vi "Acquire.vi"(8 "error in (no error)":errorcluster, 9 "Data Queue":refnum<queue>, 10 "Data Notifier":refnum<notifier>, 11 "Hardware Resources in":T1={"DO"={"task name"="AI", "task_ref"="", "lines"=""}}) -> (0 "error out":errorcluster, 3 "Hardware Resources out":T1={"DO"={"task name"="AI", "task_ref"="", "lines"=""}})   [LabVIEW 2014]
doc: "Perform the acquisition. Replace the contents of this diagram with calls to acquisition hardware."
uses:
  <vilib>/Analysis/NI_AALBase.lvlib
  <vilib>/DAQmx/read.llb/DAQmx Read (Analog 1D Wfm NChan NSamp).vi
  GLB_compteurs.vi
  PLS Digital Control.lvlib
  <vilib>/DAQmx/read.llb/DAQmx Read (Counter DBL 1Chan 1Samp).vi
  GLB_AIs.vi
  Hardware Configuration.ctl
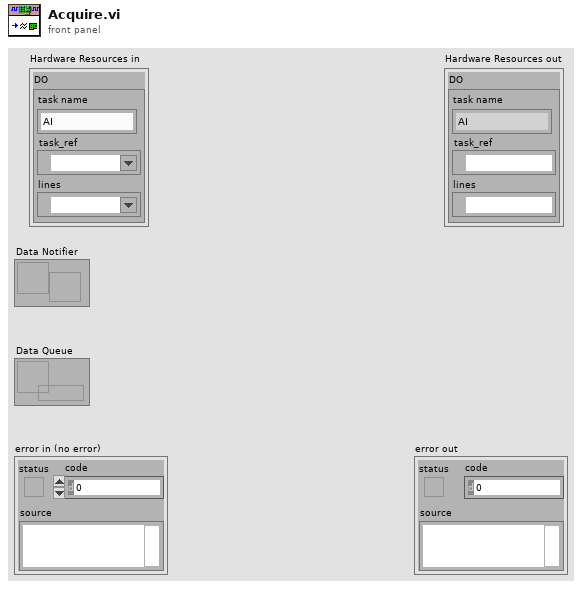
[diagram p1: front panel]
types:
  T1 = typedef "PLS Digital Control.lvlib/Hardware Configuration.ctl" = cluster{"DO":cluster{"task name":string, "task_ref":refnum<k21>, "lines":tag}}
  T2 = typedef "PLS Settings.lvlib/conversion.ctl" = cluster{"a":dbl, "b":dbl}
  T3 = cluster{"ai0":T2, "ai1":T2, "ai2":T2, "ai3":T2, "ai4":T2}
  T4 = cluster{"task name":string, "task_ref":refnum<k21>, "ctr":tag, "coeff":dbl}
  T5 = cluster{"[0]":dbl, "[1]":dbl, "[2]":dbl, "[3]":dbl, "[4]":dbl}
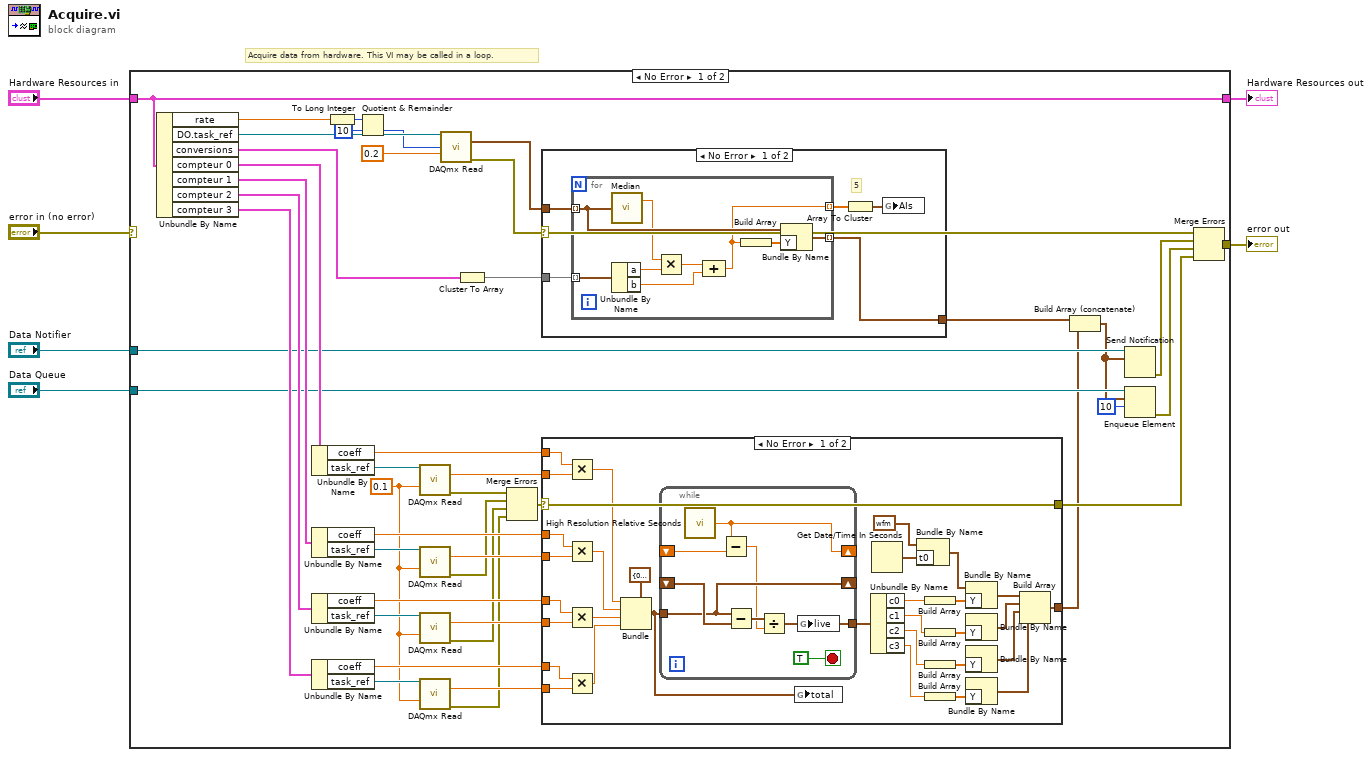
[diagram p0: block diagram]
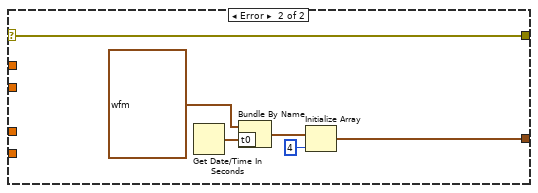
[diagram p2: hidden frame]
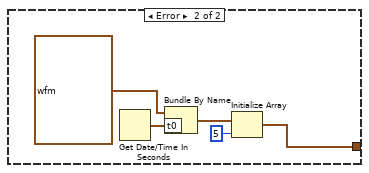
[diagram p3: hidden frame]
diagram:
  # "Acquire data from hardware. This VI may be called in a loop."
  n1 = case shown="No Error" "error in (no error)" {
    selector: "error in (no error)" -> [_ w115]
    tunnel: [w40 w115] -> w5
    tunnel: "Hardware Resources in" -> [w43 w116]
    tunnel: [w43 w116] -> w3
    tunnel: "Data Notifier" -> [w14 _]
    tunnel: "Data Queue" -> [w15 _]
    frame No Error {
      w20 = 0.1 ("timeout")
      n2 = Unbundle By Name(w43) -> ("rate"=w22:dbl, "DO.task_ref"=w49:refnum<k21>, "conversions"=w45:T3, "compteur 0"=w36:T4, "compteur 1"=w31:T4, "compteur 2"=w32:T4, "compteur 3"=w33:T4)
      n3 = Unbundle By Name(w36) -> ("coeff"=w34:dbl, "task_ref"=w35:refnum<k21>)
      n4 = Unbundle By Name(w31) -> ("coeff"=w29:dbl, "task_ref"=w30:refnum<k21>)
      n5 = Unbundle By Name(w32) -> ("coeff"=w27:dbl, "task_ref"=w28:refnum<k21>)
      n6 = Unbundle By Name(w33) -> ("coeff"=w25:dbl, "task_ref"=w26:refnum<k21>)
      n7 = To Long Integer(number=w22) -> (32bit integer=w21:i32)
      n8 = Quotient & Remainder(x=w21, y=10 ("number of samples per channel")) -> (floor(x/y)=w23:i32)  [unwired: 1 out]
      n9 = call-poly <vilib>:"DAQmx Read.vi"("task/channels in"=w35, "timeout"=w20) -> ("data"=w42:dbl, "error out"=w41:errorcluster)  [unwired: 11 in, 1 out]
      n10 = call-poly <vilib>:"DAQmx Read.vi"("task/channels in"=w30, "timeout"=w20) -> ("data"=w37:dbl, "error out"=w18:errorcluster)  [unwired: 11 in, 1 out]
      n11 = call-poly <vilib>:"DAQmx Read.vi"("task/channels in"=w28, "timeout"=w20) -> ("data"=w38:dbl, "error out"=w17:errorcluster)  [unwired: 11 in, 1 out]
      n12 = call-poly <vilib>:"DAQmx Read.vi"("task/channels in"=w26, "timeout"=w20) -> ("data"=w39:dbl, "error out"=w16:errorcluster)  [unwired: 11 in, 1 out]
      n13 = call-poly <vilib>:"DAQmx Read.vi"("task/channels in"=w49, "number of samples per channel"=w23, "timeout"=0.2) -> ("data"=w47:waveform(dbl)[], "error out"=w46:errorcluster)  [unwired: 10 in, 1 out]
      n14 = Cluster To Array(cluster=w45) -> (array=w44:T2[])
      n15 = Merge Errors(w41, w18, w17, w16) -> (w19:errorcluster)
      n16 = case shown="No Error" w46 {
        tunnel: w47 -> [w100 _]
        tunnel: w44 -> [w99 _]
        tunnel: [w96 w110] -> w13
        frame No Error {
          # "5"
          n17 = for {
            tunnel: w100 -> [w109] mode=indexing
            tunnel: [w108] -> w96 mode=indexing
            tunnel: w99 -> [w107] mode=indexing
            tunnel: [w101] -> w98 mode=indexing
            n18 = call <vilib>:"Median.vi"("X"=w109) -> ("median"=w105:dbl)  [unwired: 1 out]
            n19 = Unbundle By Name(w107) -> ("a"=w106:dbl, "b"=w103:dbl)
            n20 = Multiply(x=w105, y=w106) -> (x*y=w104:dbl)
            n21 = Compound Arithmetic op=ADD(w104, w103) -> (w101:dbl)
            n22 = Build Array(w101) -> (w102:dbl[])
            n23 = Bundle By Name(cluster=w109, "Y"=w102) -> (w108:waveform(dbl))
          }
          n24 = Array To Cluster(array=w98) -> (cluster=w97:T5)
          n25 = global write "GLB_AIs.vi" "AIs"(w97) -> ()
        }
        frame Error {
          n26 = Get Date/Time In Seconds() -> (seconds since 1Jan1904=w114:timestamp)
          n27 = Bundle By Name(cluster=waveform(dbl) {"t0"=timestamp(0 s since 1904-01-01), "dt"=0.1, "Y"=[nan]} ("waveform"), "t0"=w114) -> (w112:waveform(dbl))
          n28 = Initialize Array(w112, 5 ("dimension size")) -> (w110:waveform(dbl)[])
        }
      }
      n29 = case shown="No Error" w19 {
        selector: w19 -> [w80 w95]
        tunnel: w42 -> [w81 _]
        tunnel: w34 -> [w76 _]
        tunnel: [w80 w95] -> w12
        tunnel: w39 -> [w79 _]
        tunnel: w38 -> [w78 _]
        tunnel: w37 -> [w77 _]
        tunnel: w29 -> [w72 _]
        tunnel: w27 -> [w71 _]
        tunnel: w25 -> [w70 _]
        tunnel: [w50 w90] -> w7
        frame No Error {
          n30 = Multiply(x=w76, y=w81) -> (x*y=w66:dbl)
          n31 = Multiply(x=w72, y=w77) -> (x*y=w75:dbl)
          n32 = Multiply(x=w71, y=w78) -> (x*y=w74:dbl)
          n33 = Multiply(x=w70, y=w79) -> (x*y=w73:dbl)
          n34 = Bundle(cluster=cluster{"c0":dbl, "c1":dbl, "c2":dbl, "c3":dbl} {"c0"=0.0, "c1"=0.0, "c2"=0.0, "c3"=0.0} ("live"), "c0"=w66, "c1"=w75, "c2"=w74, "c3"=w73) -> (w69:cluster{"c0":dbl, "c1":dbl, "c2":dbl, "c3":dbl})
          n35 = while {
            tunnel: w69 -> [w87]
            shift-right: [w87] -> _
            shift-left: _ -> [w88]
            shift-right: [w85] -> _
            shift-left: _ -> [w84]
            tunnel: [w82] -> w68
            stop <- TRUE stop-if-true
            n36 = call <vilib>:"High Resolution Relative Seconds.vi"() -> ("relative seconds"=w85:dbl)
            n37 = Subtract(x=w85, y=w84) -> (x-y=w83:dbl)
            n38 = Subtract(x=w87, y=w88) -> (x-y=w86:cluster{"c0":dbl, "c1":dbl, "c2":dbl, "c3":dbl})
            n39 = Divide(x=w86, y=w83) -> (x/y=w82:cluster{"c0":dbl, "c1":dbl, "c2":dbl, "c3":dbl})
            n40 = global write "GLB_compteurs.vi" "live"(w82) -> ()
          }
          n41 = global write "GLB_compteurs.vi" "total"(w69) -> ()
          n42 = Unbundle By Name(w68) -> ("c0"=w64:dbl, "c1"=w54:dbl, "c2"=w55:dbl, "c3"=w56:dbl)
          n43 = Get Date/Time In Seconds() -> (seconds since 1Jan1904=w65:timestamp)
          n44 = Bundle By Name(cluster=waveform(dbl) {"t0"=timestamp(0 s since 1904-01-01), "dt"=0.1, "Y"=[]} ("waveform"), "t0"=w65) -> (w62:waveform(dbl))
          n45 = Build Array(w64) -> (w61:dbl[])
          n46 = Build Array(w54) -> (w59:dbl[])
          n47 = Build Array(w55) -> (w58:dbl[])
          n48 = Build Array(w56) -> (w57:dbl[])
          n49 = Bundle By Name(cluster=w62, "Y"=w61) -> (w60:waveform(dbl))
          n50 = Bundle By Name("Y"=w59) -> (w53:waveform(dbl))  [unwired: 1 in]
          n51 = Bundle By Name("Y"=w58) -> (w52:waveform(dbl))  [unwired: 1 in]
          n52 = Bundle By Name("Y"=w57) -> (w51:waveform(dbl))  [unwired: 1 in]
          n53 = Build Array(w60, w53, w52, w51) -> (w50:waveform(dbl)[])
        }
        frame Error {
          n54 = Get Date/Time In Seconds() -> (seconds since 1Jan1904=w94:timestamp)
          n55 = Bundle By Name(cluster=waveform(dbl) {"t0"=timestamp(0 s since 1904-01-01), "dt"=0.1, "Y"=[nan]} ("waveform"), "t0"=w94) -> (w92:waveform(dbl))
          n56 = Initialize Array(w92, 4 ("dimension size")) -> (w90:waveform(dbl)[])
        }
      }
      n57 = Build Array (concatenate)(w13, w7) -> (w9:waveform(dbl)[])
      n58 = Send Notification(notification=w9, notifier=w14) -> (error out=w11:errorcluster)  [unwired: 1 in, 1 out]
      n59 = Enqueue Element(queue=w15, element=w9, timeout in ms (-1)=10) -> (error out=w10:errorcluster)  [unwired: 1 in, 2 out]
      n60 = Merge Errors(w46, w11, w10, w12) -> (w40:errorcluster)
    }
    frame Error {
    }
  }
  "Hardware Resources out" <- w3
  "error out" <- w5
